vi "FlatToRichgoogle_protobuf_Enum.vi"(5 "OutputClusterType":T1, 11 "InputCluster":T7) -> (3 "OutputCluster":T1)   [LabVIEW 2020, in "Measurement Plugin Measurement Server Internal.lvlib"]
uses:
  Measurement Plugin Measurement Server Internal.lvlib
  google_protobuf_Enum_Flat.ctl
  google_protobuf_EnumValue_Flat.ctl
  google_protobuf_Option_Flat.ctl
  google_protobuf_Any_Flat.ctl
  google_protobuf_SourceContext_Flat.ctl
  google_protobuf_Syntax.ctl
  google_protobuf_Enum.ctl
  google_protobuf_EnumValue.ctl
  google_protobuf_Option.ctl
  google_protobuf_Any.ctl
  google_protobuf_SourceContext.ctl
  FlatToRichgoogle_protobuf_Any.vi
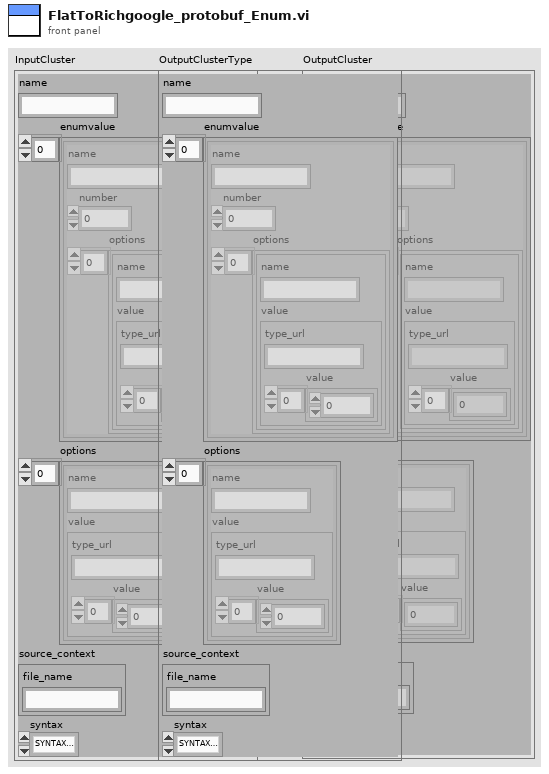
[diagram p1: front panel]
types:
  T1 = typedef "Measurement Plugin Measurement Server Internal.lvlib/google_protobuf_Enum.ctl" = cluster{"name":string, "enumvalue":T2[], "options":T3[], "source_context":T5, "syntax":T6}
  T2 = typedef "Measurement Plugin Measurement Server Internal.lvlib/google_protobuf_EnumValue.ctl" = cluster{"name":string, "number":i32, "options":T3[]}
  T3 = typedef "Measurement Plugin Measurement Server Internal.lvlib/google_protobuf_Option.ctl" = cluster{"name":string, "value":T4}
  T4 = typedef "Measurement Plugin Measurement Server Internal.lvlib/google_protobuf_Any.ctl" = cluster{"type_url":string, "value":u8[]}
  T5 = typedef "Measurement Plugin Measurement Server Internal.lvlib/google_protobuf_SourceContext.ctl" = cluster{"file_name":string}
  T6 = typedef "Measurement Plugin Measurement Server Internal.lvlib/google_protobuf_Syntax.ctl" = enum32{"SYNTAX_PROTO2", "SYNTAX_PROTO3"}
  T7 = typedef "Measurement Plugin Measurement Server Internal.lvlib/google_protobuf_Enum_Flat.ctl" = cluster{"name":string, "enumvalue":T8[], "options":T9[], "source_context":T11, "syntax":T6}
  T8 = typedef "Measurement Plugin Measurement Server Internal.lvlib/google_protobuf_EnumValue_Flat.ctl" = cluster{"name":string, "number":i32, "options":T9[]}
  T9 = typedef "Measurement Plugin Measurement Server Internal.lvlib/google_protobuf_Option_Flat.ctl" = cluster{"name":string, "value":T10}
  T10 = typedef "Measurement Plugin Measurement Server Internal.lvlib/google_protobuf_Any_Flat.ctl" = cluster{"type_url":string, "value":u8[]}
  T11 = typedef "Measurement Plugin Measurement Server Internal.lvlib/google_protobuf_SourceContext_Flat.ctl" = cluster{"file_name":string}
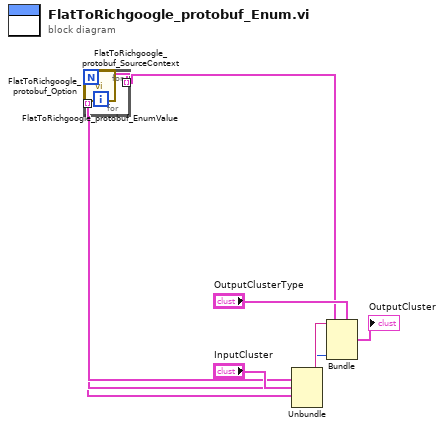
[diagram p0: block diagram]
diagram:
  n1 = Unbundle "Unbundle"("InputCluster") -> ("name"=w8:string, "enumvalue"=w7:T8[], "options"=w5:T9[], "source_context"=w3:T11, "syntax"=w1:T6)
  n2 = call "FlatToRichgoogle_protobuf_SourceContext.vi"("InputCluster"=w3) -> ("OutputCluster"=w2:T5)  [unwired: 10 in]
  n3 = for {
    tunnel: w5 -> [w13] mode=indexing
    tunnel: [w12] -> w4 mode=indexing
    n4 = call "FlatToRichgoogle_protobuf_Option.vi"("InputCluster"=w13) -> ("OutputCluster"=w12:T3)  [unwired: 10 in]
  }
  n5 = for {
    tunnel: w7 -> [w15] mode=indexing
    tunnel: [w14] -> w6 mode=indexing
    n6 = call "FlatToRichgoogle_protobuf_EnumValue.vi"("InputCluster"=w15) -> ("OutputCluster"=w14:T2)  [unwired: 10 in]
  }
  n7 = Bundle "Bundle"(cluster="OutputClusterType", "name"=w8, "enumvalue"=w6, "options"=w4, "source_context"=w2, "syntax"=w1) -> (→"OutputCluster":T1)
